vi "ABB configure Noise test.vi"() -> ()   [LabVIEW 2017]
uses:
  ABB global.vi
panel:
  out "Image File":string
  in  "Type Select":T1
  in  "Noise Test Images":i32(listbox)
  in  "Edit Types":T2
  out "Picture":picture
  in  "Exit":bool
  # "Configure Noise Test"
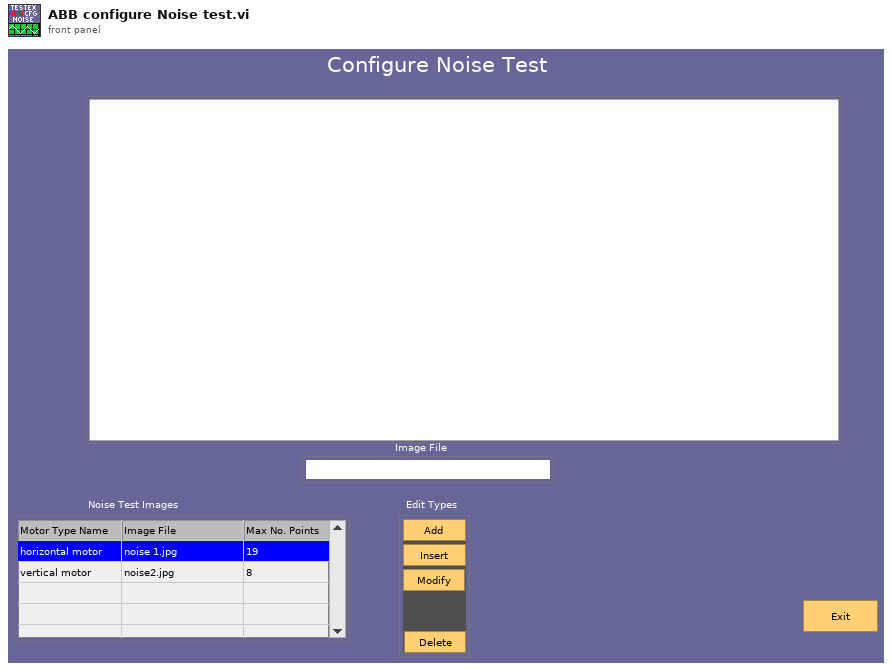
[diagram p1: front panel]
types:
  T1 = cluster{" Type Name":string, "Select Image":bool, "OK":bool, "Cancel":bool, "No. Points":i32}
  T2 = cluster{"Add":bool, "Insert":bool, "Delete":bool, "modify":bool}
  T3 = enum32{"existing file", "new file", "new or existing file", "existing dir", "new dir", "new or existing dir", "existing file (use LLBs)", "new file (use LLBs)", "new or existing file (use LLBs)", "new or existing file or directory (use LLBs)"}
  T4 = typedef "imagedata.ctl" = cluster{"image type":i32, "image depth":i32, "image":u8[], "mask":u8[], "colors":u32[], "Rectangle":cluster{"left":i16, "top":i16, "right":i16, "bottom":i16}}
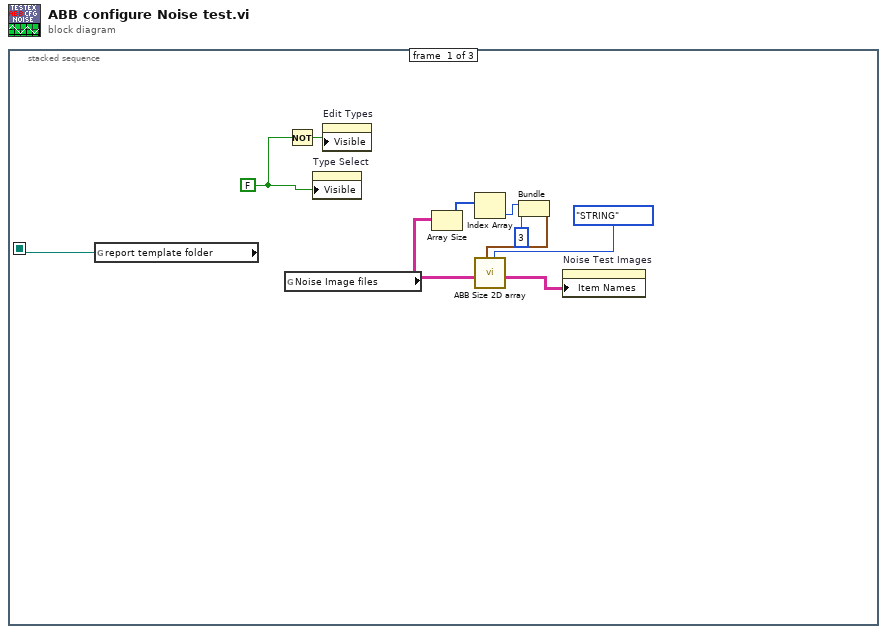
[diagram p0: block diagram]
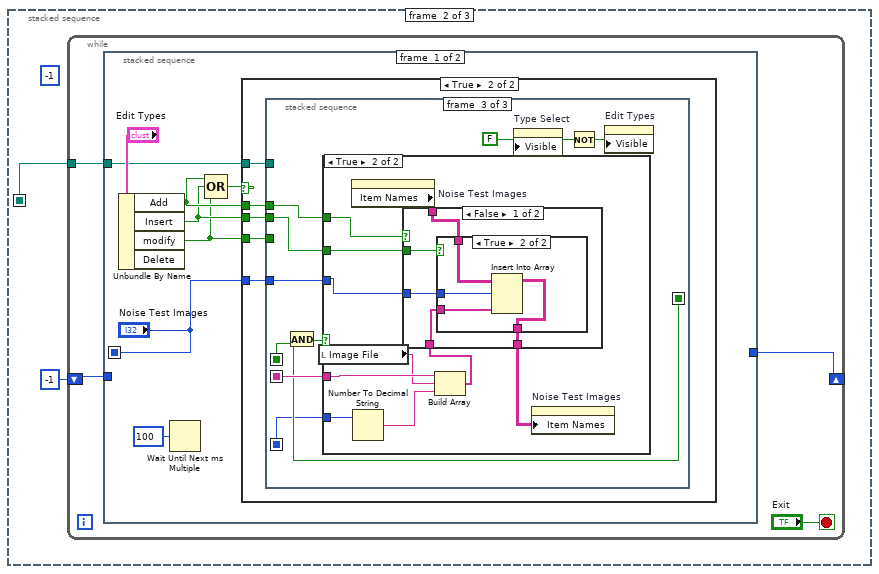
[diagram p2: hidden frame]
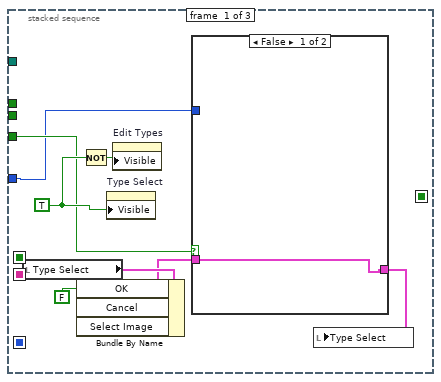
[diagram p4: hidden frame]
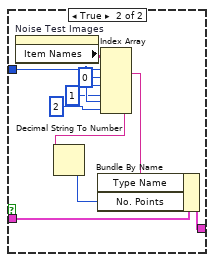
[diagram p5: hidden frame]
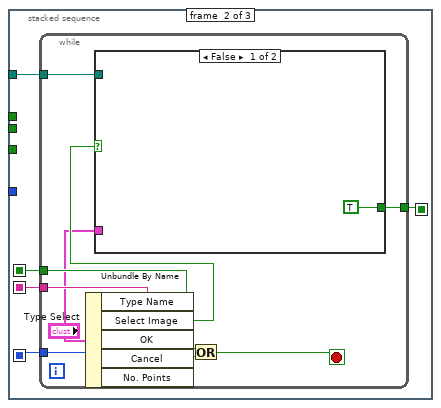
[diagram p6: hidden frame]
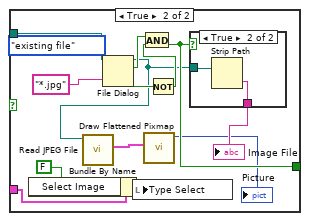
[diagram p7: hidden frame]
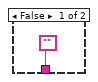
[diagram p8: hidden frame]
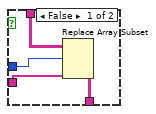
[diagram p10: hidden frame]
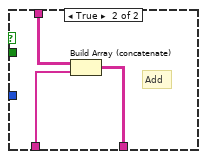
[diagram p11: hidden frame]
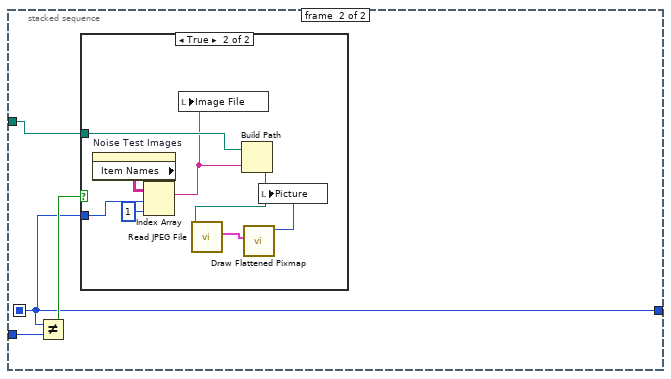
[diagram p12: hidden frame]
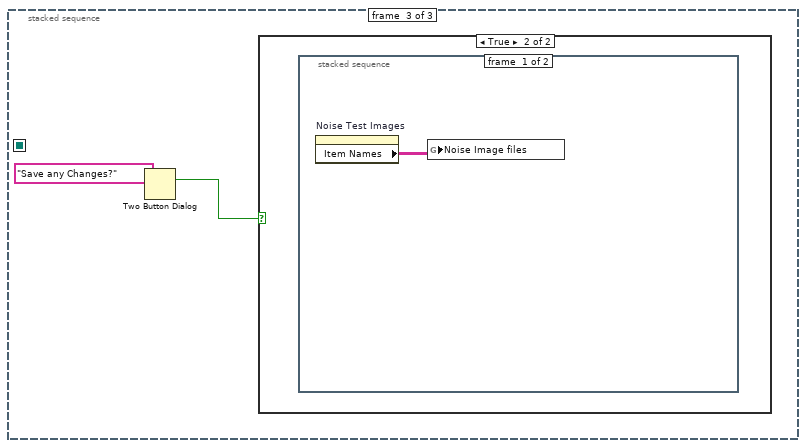
[diagram p14: hidden frame]
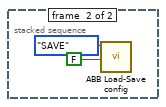
[diagram p16: hidden frame]
diagram:
  n1 = stacked-sequence {
    seq-local: [w8 _ _] -> [_ w12 _]
    frame #0 {
      w10 = FALSE ("Visible")
      n2 = global read "ABB global.vi" "report template folder"() -> (w8:path)
      n3 = global read "ABB global.vi" "Noise Image files"() -> (w7:string[][])
      n4 = Not(x=w10) -> (.not. x?=w9:bool)
      n5 = property on="Type Select" class="Clust (strict)"("Visible"=w10) -> ()  [unwired: 2 in, 2 out]
      n6 = property on="Edit Types" class="Clust"("Visible"=w9) -> ()  [unwired: 2 in, 2 out]
      n7 = Array Size(array=w7) -> (size(s)=w5:i32[])
      n8 = Index Array(array=w5) -> (element=w4:i32)  [unwired: 1 in]
      n9 = Bundle(w4, 3) -> (w2:cluster{i32, i32})  [unwired: 1 in]
      n10 = call "ABB Size 2D array.vi"("Type"=enum16{"Integer", "DBL", "STRING", "BOOLEAN"}."STRING", "Size"=w2, "String Array in"=w7) -> ("String Array out"=w6:string[][])  [unwired: 5 in, 3 out]
      n11 = property on="Noise Test Images" class="MCListbox (strict)"("Item Names"=w6) -> ()  [unwired: 2 in, 2 out]
    }
    frame #1 {
      (unwired) -1 ("Number Values")
      n12 = while {
        tunnel: w12 -> [w15]
        shift-right: [w14] -> _
        shift-left: -1 ("Noise Test Images") -> [w13]
        stop <- "Exit" stop-if-true
        n13 = stacked-sequence {
          seq-local: ["Noise Test Images" _] -> [_ w117]
          tunnel: w15 -> [w21 w116]
          tunnel: [_ w117] -> w14
          tunnel: w13 -> [_ w119]
          frame #0 {
            n14 = Unbundle By Name("Edit Types") -> ("Add"=w20:bool, "Insert"=w19:bool, "modify"=w17:bool)  [unwired: 1 out]
            n15 = Wait Until Next ms Multiple(millisecond multiple=u32 100) -> ()  [unwired: 1 out]
            n16 = Compound Arithmetic op=OR(w20, w19, w17) -> (w22:bool)
            n17 = case shown="True" w22 {
              tunnel: w21 -> [_ w29]
              tunnel: "Noise Test Images" -> [_ w28]
              tunnel: w20 -> [_ w27]
              tunnel: w19 -> [_ w26]
              tunnel: w17 -> [_ w25]
              frame False {
              }
              frame True {
                n18 = stacked-sequence {
                  seq-local: [_ w53 _] -> [_ _ w87]
                  seq-local: [_ w51 _] -> [_ _ w86]
                  seq-local: [_ w49 _] -> [_ _ w81]
                  seq-local: [_ w50 _] -> [_ _ w80]
                  tunnel: w29 -> [_ w52 _]
                  tunnel: w28 -> [w34 _ w85]
                  tunnel: w27 -> [_ _ w84]
                  tunnel: w26 -> [_ _ w83]
                  tunnel: w25 -> [w35 _ _]
                  frame #0 {
                    w30 = FALSE
                    w37 = TRUE ("Visible")
                    n19 = local read "Type Select"() -> (w32:T1)
                    n20 = Bundle By Name(cluster=w32, "OK"=w30, "Cancel"=w30, "Select Image"=w30) -> (w31:T1)
                    n21 = Not(x=w37) -> (.not. x?=w36:bool)
                    n22 = property on="Type Select" class="Clust (strict)"("Visible"=w37) -> ()  [unwired: 2 in, 2 out]
                    n23 = property on="Edit Types" class="Clust"("Visible"=w36) -> ()  [unwired: 2 in, 2 out]
                    n24 = case shown="False" w35 {
                      tunnel: w34 -> [_ w47]
                      tunnel: w31 -> [w38 w40]
                      tunnel: [w38 w39] -> w33
                      frame False {
                      }
                      frame True {
                        n25 = property on="Noise Test Images" class="MCListbox (strict)"() -> ("Item Names"=w48:string[][])  [unwired: 2 in, 2 out]
                        n26 = Index Array(array=w48, index (row) #1=w47, index (col) #1=0 ("disabled index (col)"), index (row) #2=w47, index (col) #2=1 ("disabled index (col)"), index (row) #3=w47, index (col) #3=2 ("disabled index (col)")) -> (element #1=w43:string, element #3=w42:string)  [unwired: 1 out]
                        n27 = Decimal String To Number(string=w42) -> (number=w41:i32)  [unwired: 2 in, 1 out]
                        n28 = Bundle By Name(cluster=w40, "Type Name"=w43, "No. Points"=w41) -> (w39:T1)
                      }
                    }
                    n29 = local write "Type Select"(w33) -> ()
                  }
                  frame #1 {
                    n30 = while {
                      tunnel: [w60] -> w53
                      tunnel: w52 -> [w58]
                      tunnel: [w57] -> w51
                      tunnel: [w56] -> w50
                      tunnel: [w54] -> w49
                      stop <- w61 stop-if-true
                      n31 = Unbundle By Name("Type Select") -> ("Type Name"=w57:string, "Select Image"=w59:bool, "OK"=w60:bool, "Cancel"=w62:bool, "No. Points"=w56:i32)
                      n32 = case shown="False" w59 {
                        tunnel: w58 -> [_ w75]
                        tunnel: [TRUE w70] -> w54
                        tunnel: "Type Select" -> [_ w66]
                        frame False {
                        }
                        frame True {
                          (unwired) T3."existing file" ("select mode (2)")
                          n33 = Bundle By Name(cluster=w66, "Select Image"=FALSE) -> (w65:T1)
                          n34 = File Dialog(6:"*.jpg" ("pattern"), 11:w75) -> (1:w73:bool, 2:w74:bool, 3:w69:path)  [unwired: 5 in, 1 out]
                          n35 = call <vilib>:"Read JPEG File.vi"("path to JPEG file"=w69) -> ("image data"=w68:T4)  [unwired: 8 in, 2 out]
                          n36 = local write "Type Select"(w65) -> ()
                          n37 = call <vilib>:"Draw Flattened Pixmap.vi"("image data"=w68) -> ("new picture"=→"Picture":picture)  [unwired: 8 in]
                          n38 = Not(x=w73) -> (.not. x?=w72:bool)
                          n39 = And(x=w74, y=w72) -> (x .and. y?=w70:bool)
                          n40 = case shown="True" w70 {
                            tunnel: w69 -> [_ w79]
                            tunnel: ["" w78] -> w71
                            frame False {
                            }
                            frame True {
                              n41 = Strip Path(path=w79) -> (name=w78:string)  [unwired: 1 out]
                            }
                          }
                          "Image File" <- w71
                        }
                      }
                      n42 = Or(x=w60, y=w62) -> (x .or. y?=w61:bool)
                    }
                  }
                  frame #2 {
                    w89 = FALSE ("Visible")
                    n43 = And(x=w81, y=w87) -> (x .and. y?=w82:bool)
                    n44 = case shown="True" w82 {
                      tunnel: w86 -> [_ w96]
                      tunnel: w85 -> [_ w92]
                      tunnel: w84 -> [_ w99]
                      tunnel: w83 -> [_ w93]
                      tunnel: w80 -> [_ w91]
                      frame False {
                      }
                      frame True {
                        n45 = local read "Image File"() -> (w95:string)
                        n46 = property on="Noise Test Images" class="MCListbox (strict)"() -> ("Item Names"=w98:string[][])  [unwired: 2 in, 2 out]
                        n47 = Number To Decimal String(number=w91) -> (decimal integer string=w90:string)  [unwired: 1 in]
                        n48 = Build Array(w96, w95, w90) -> (w94:string[])
                        n49 = case shown="False" w99 {
                          tunnel: w98 -> [w103 w115]
                          tunnel: [w101 w113] -> w97
                          tunnel: w94 -> [w100 w114]
                          tunnel: w93 -> [w104 _]
                          tunnel: w92 -> [w102 _]
                          frame False {
                            n50 = case shown="True" w104 {
                              tunnel: w103 -> [w108 w112]
                              tunnel: w102 -> [w107 w111]
                              tunnel: [w105 w110] -> w101
                              tunnel: w100 -> [w106 w109]
                              frame False {
                                n51 = Replace Array Subset "Replace Array Subset"(array=w108, new element=w106, index (row)=w107) -> (w105:string[][])  [unwired: 1 in]
                              }
                              frame True {
                                n52 = Insert Into Array "Insert Into Array"(array=w112, index (row)=w111, new element=w109) -> (w110:string[][])  [unwired: 1 in]
                              }
                            }
                          }
                          frame True {
                            # "Add"
                            n53 = Build Array (concatenate)(w115, w114) -> (w113:string[][])
                          }
                        }
                        n54 = property on="Noise Test Images" class="MCListbox (strict)"("Item Names"=w97) -> ()  [unwired: 2 in, 2 out]
                      }
                    }
                    n55 = property on="Type Select" class="Clust (strict)"("Visible"=w89) -> ()  [unwired: 2 in, 2 out]
                    n56 = Not(x=w89) -> (.not. x?=w88:bool)
                    n57 = property on="Edit Types" class="Clust"("Visible"=w88) -> ()  [unwired: 2 in, 2 out]
                  }
                }
              }
            }
          }
          frame #1 {
            n58 = Not Equal?(x=w117, y=w119) -> (x != y?=w118:bool)
            n59 = case shown="True" w118 {
              tunnel: w117 -> [_ w126]
              tunnel: w116 -> [_ w124]
              frame False {
              }
              frame True {
                n60 = property on="Noise Test Images" class="MCListbox (strict)"() -> ("Item Names"=w127:string[][])  [unwired: 2 in, 2 out]
                n61 = Index Array(array=w127, index (row)=w126, index (col)=1 ("disabled index (col)")) -> (element=w120:string)
                n62 = local write "Image File"(w120) -> ()
                n63 = Build Path(base path=w124, name or relative path=w120) -> (appended path=w122:path)
                n64 = call <vilib>:"Read JPEG File.vi"("path to JPEG file"=w122) -> ("image data"=w123:T4)  [unwired: 8 in, 2 out]
                n65 = call <vilib>:"Draw Flattened Pixmap.vi"("image data"=w123) -> ("new picture"=w121:picture)  [unwired: 8 in]
                n66 = local write "Picture"(w121) -> ()
              }
            }
          }
        }
      }
    }
    frame #2 {
      n67 = Two Button Dialog(message="Save any Changes?") -> (T button?=w129:bool)  [unwired: 2 in]
      n68 = case shown="True" w129 {
        frame False {
        }
        frame True {
          n69 = stacked-sequence {
            frame #0 {
              n70 = property on="Noise Test Images" class="MCListbox (strict)"() -> ("Item Names"=w130:string[][])  [unwired: 2 in, 2 out]
              n71 = global write "ABB global.vi" "Noise Image files"(w130) -> ()
            }
            frame #1 {
              n72 = call "ABB Load-Save config.vi"("confirm save"=FALSE, "Mode"=enum16{"LOAD", "SAVE"}."SAVE") -> ()  [unwired: 10 in]
            }
          }
        }
      }
    }
  }
